vi "2DGaussianRotationModel2.vi"(3 "output control":T1, 4 "data":T2, 5 "X":dbl[](array[numeric]), 6 "a":dbl[](array[numeric])) -> (0 "error out":errorcluster, 1 "f'(X,a)":dbl[][](array[numeric]), 2 "f(X,a)":dbl[](array[numeric]))   [LabVIEW 2012]
doc: "This template is the starting point for creating a model function to be passed to the Nonlinear Curve Fit.vi."
uses:
  <vilib>/gmath/NumericalOptimization/objective function data.ctl
  <vilib>/gmath/NumericalOptimization/LM_output select.ctl
  <vilib>/Analysis/Matrix/Numeric/Conversions/Array To Matrix - RA2.vi
  <vilib>/Analysis/baseanly.llb/A x Vector.vi
  <vilib>/Analysis/NI_AALBase.lvlib
  <vilib>/Analysis/Matrix/NI_Matrix.lvlib
  <vilib>/gmath/NI_Gmath.lvlib
panel:
  out "Height":i32
  out "Width":i32
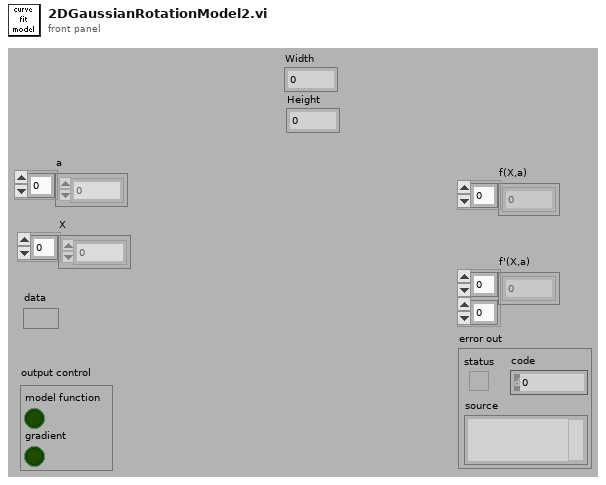
[diagram p1: front panel]
types:
  T1 = typedef "NI_Gmath.lvlib/LM_output select.ctl" = cluster{"model function":bool, "gradient":bool}
  T2 = typedef "NI_Gmath.lvlib/objective function data.ctl" = variant
  T3 = cluster{"XScale.Maximum":dbl, "YScale.Maximum":dbl}
  T4 = typedef "NI_Matrix.lvlib/RealMatrix.ctl" = dbl[][]
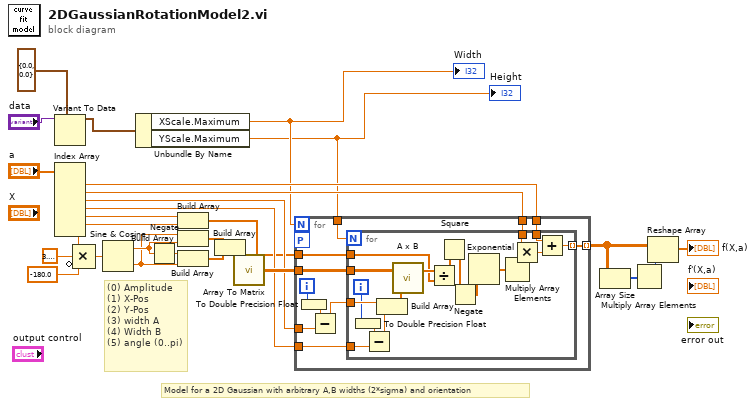
[diagram p0: block diagram]
diagram:
  # "Model for a 2D Gaussian with arbitrary A,B widths (2*sigma) and orientation"
  # "(0) Amplitude\n(1) X-Pos\n(2) Y-Pos\n(3) width A\n(4) Width B\n(5) angle (0..pi)"
  n1 = Variant To Data(type=T3 {"XScale.Maximum"=0.0, "YScale.Maximum"=0.0}, Variant="data") -> (data=w3:T3)  [unwired: 1 in, 1 out]
  n2 = Index Array(array="a") -> (element #1=w5:dbl, element #2=w18:dbl, element #3=w12:dbl, element #4=w11:dbl, element #5=w17:dbl, element #6=w16:dbl, element #7=w10:dbl)  [unwired: 7 in]
  n3 = Compound Arithmetic op=MULTIPLY(w10, 3.141592653589793, invert -180.0 ("value")) -> (w9:dbl)
  n4 = Sine & Cosine(0:w9) -> (1:w27:dbl, 2:w26:dbl)
  n5 = Unbundle By Name(w3) -> ("XScale.Maximum"=w2:dbl, "YScale.Maximum"=w1:dbl)
  "Width" <- w2
  "Height" <- w1
  n6 = Negate(x=w27) -> (-x=w28:dbl)
  n7 = Build Array(w17, w16) -> (w6:dbl[])
  n8 = Build Array(w26, w27) -> (w25:dbl[])
  n9 = Build Array(w28, w26) -> (w24:dbl[])
  n10 = Build Array(w25, w24) -> (w23:dbl[][])
  n11 = call-poly <vilib>:"Array To Matrix.vi"("Real 2D Array"=w23) -> ("Real Matrix"=w22:T4)
  n12 = for {
    N: w2 -> [_]
    tunnel: w22 -> [w39]
    tunnel: w6 -> [w38]
    tunnel: [w37] -> w21 mode=indexing
    tunnel: w18 -> [w36]
    tunnel: w1 -> [w35]
    tunnel: w12 -> [w32]
    tunnel: w11 -> [w30]
    workers-P: _ -> [_]
    tunnel: w5 -> [w29]
    i -> [w34]
    n13 = To Double Precision Float(number=w34) -> (double precision float=w33:dbl)
    n14 = Subtract(x=w33, y=w32) -> (x-y=w31:dbl)
    n15 = for {
      N: w35 -> [_]
      tunnel: w31 -> [w57]
      tunnel: w39 -> [w55]
      tunnel: w38 -> [w53]
      tunnel: [w41] -> w37 mode=indexing
      tunnel: w36 -> [w50]
      tunnel: w30 -> [w47]
      tunnel: w29 -> [w40]
      i -> [w49]
      n16 = To Double Precision Float(number=w49) -> (double precision float=w48:dbl)
      n17 = Subtract(x=w48, y=w47) -> (x-y=w46:dbl)
      n18 = Build Array(w57, w46) -> (w56:dbl[])
      n19 = call-poly <vilib>:"A x B.vi"("Vector"=w56, "A"=w55) -> ("A x Vector"=w54:dbl[])  [unwired: 1 out]
      n20 = Divide(x=w54, y=w53) -> (x/y=w45:dbl[])
      n21 = Square(x=w45) -> (x^2=w44:dbl[])
      n22 = Negate(x=w44) -> (-x=w43:dbl[])
      n23 = Exponential(1:w43) -> (0:w52:dbl[])
      n24 = Multiply Array Elements(1:w52) -> (0:w51:dbl)
      n25 = Multiply(x=w50, y=w51) -> (x*y=w42:dbl)
      n26 = Add(x=w40, y=w42) -> (x+y=w41:dbl)
    }
  }
  n27 = Array Size(array=w21) -> (size(s)=w19:i32[])
  n28 = Multiply Array Elements(1:w19) -> (0:w20:i32)
  n29 = Reshape Array(w21, w20) -> (→"f(X,a)":dbl[])
